vi "ReadHTTPMethod.vi"(11 "Method":T2) -> (2 "HTTP method_NET":T1, 3 "HTTP method":T2)   [LabVIEW 2018, in "REST Client_NET.lvlib" / "REST Client_NET.lvclass"]
doc: "<b> </b> <b> </b>\nHttpClient_NET\nJustin Young - Viviota\nCopyright (c) 2021\nLicense: BSD"
uses:
  REST Client_NET.lvclass
  classes/REST Client/HTTP Methods.ctl
  Types/method_enum.ctl
  HttpClient_NET.lvlib
  classes/REST Client/REST Client.lvclass
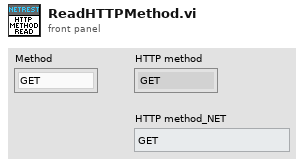
[diagram p1: front panel]
types:
  T1 = typedef "HttpClient_NET.lvlib/method_enum.ctl" = enum16{"GET", "PUT", "POST", "DELETE", "HEAD", "TRACE", "SEND"}
  T2 = typedef "REST Client_JKI.lvlib/REST Client.lvclass/HTTP Methods.ctl" = enum16{"GET", "HEAD", "POST", "PUT", "DELETE"}
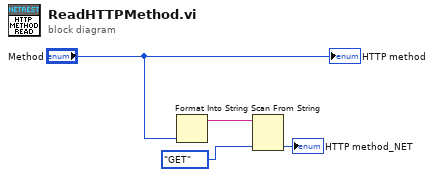
[diagram p0: block diagram]
diagram:
  n1 = Format Into String("Method") -> (resulting string=w3:string)  [unwired: 3 in, 1 out]
  n2 = Scan From String(input string=w3, default 1=method_enum."GET" ("Method")) -> (output 1=→"HTTP method_NET":T1)  [unwired: 3 in, 3 out]
  "HTTP method" <- "Method"
